vi "DEMO.vi"() -> ()   [LabVIEW 2013]
uses:
  NYPizzaStore.lvclass/NYPizzaStore.lvclass
  ChicagoPizzaStore.lvclass/ChicagoPizzaStore.lvclass
  PizzaStore.lvclass/PizzaStore.lvclass
panel:
  out "Array":string[](array[string])
  # "抽象工廠模式簡例\n\n紐約與芝加哥比薩店"
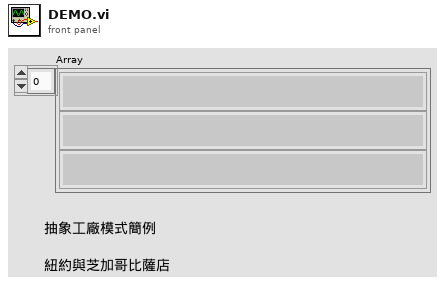
[diagram p1: front panel]
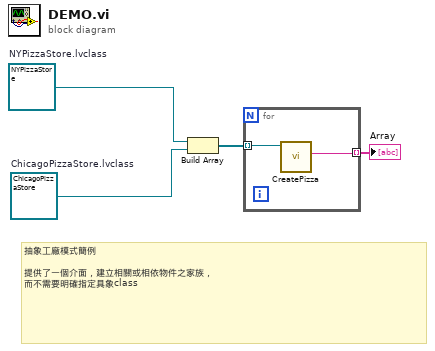
[diagram p0: block diagram]
diagram:
  w3 = refnum<class "ChicagoPizzaStore.lvclass"> refnum  # ChicagoPizzaStore.lvclass
  w4 = refnum<class "NYPizzaStore.lvclass"> refnum  # NYPizzaStore.lvclass
  # "抽象工廠模式簡例\n\n提供了一個介面，建立相關或相依物件之家族，\n而不需要明確指定具象class"
  n1 = Build Array(w4, w3) -> (w2:refnum<class "PizzaStore.lvclass">[])
  n2 = for {
    tunnel: w2 -> [w6] mode=indexing
    tunnel: [w5] -> w1 mode=indexing
    n3 = call-dynamic "CreatePizza.vi"("PizzaStore in"=w6) -> ("Pizza"=w5:string)  [unwired: 8 in, 2 out]
  }
  "Array" <- w1
